vi "Validate move.vi"(7 "Position":refnum<class "Position.lvclass">, 9 "Destination":T1={"File"=enum."d", "Rank"=enum."4"}, 10 "Source":T1={"File"=enum."d", "Rank"=enum."4"}) -> (2 "Valid move":bool, 3 "Move":refnum<class "Move.lvclass">)   [LabVIEW 2016, in "Chesslib.lvlib" / "Move.lvclass"]
uses:
  Move.lvclass
  Pieces/Piece/Piece.lvclass
  Position/Position.lvclass
  typedef/Rank.ctl
  Chesslib.lvlib
  typedef/File.ctl
  typedef/Square.ctl
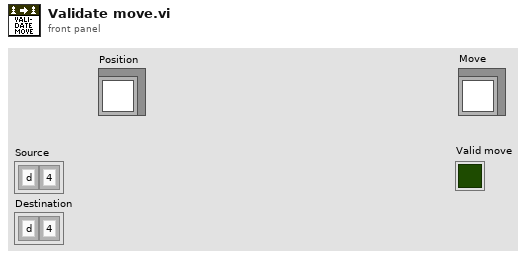
[diagram p1: front panel]
types:
  T1 = typedef "Chesslib.lvlib/Square.ctl" = cluster{"File":T2, "Rank":T3}
  T2 = typedef "Chesslib.lvlib/File.ctl" = enum8{"a", "b", "c", "d", "e", "f", "g", "h"}
  T3 = typedef "Chesslib.lvlib/Rank.ctl" = enum8{"1", "2", "3", "4", "5", "6", "7", "8"}
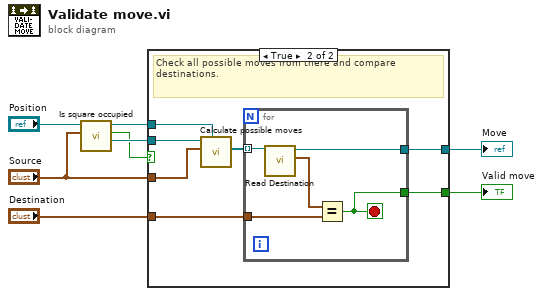
[diagram p0: block diagram]
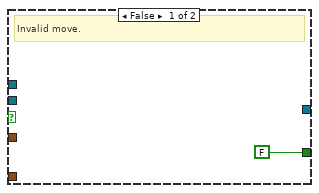
[diagram p2: hidden frame]
diagram:
  n1 = call "Is square occupied.vi"("Square"="Source", "Position in"="Position") -> ("Piece"=w2:refnum<class "Piece.lvclass">, "Occupied"=w1:bool, "Position out"=w4:refnum<class "Position.lvclass">)  [unwired: 6 in, 1 out]
  n2 = case shown="True" w1 {
    tunnel: "Source" -> [_ w16]
    tunnel: "Destination" -> [_ w15]
    tunnel: [_ w14] -> w6
    tunnel: [FALSE w13] -> w5
    tunnel: w4 -> [_ w11]
    tunnel: w2 -> [_ w10]
    frame False {
      # "Invalid move."
    }
    frame True {
      # "Check all possible moves from there and compare destinations."
      n3 = call "Calculate possible moves.vi"("Position"=w11, "Source"=w16, "Piece in"=w10) -> ("Moves"=w12:refnum<class "Move.lvclass">[])  [unwired: 6 in, 2 out]
      n4 = for {
        tunnel: w12 -> [w17] mode=indexing
        tunnel: w15 -> [w21]
        tunnel: [w19] -> w13
        tunnel: [w18] -> w14
        stop <- w19 stop-if-true
        n5 = call "Read Destination.vi"("Move in"=w17) -> ("Square"=w20:T1, "Move out"=w18:refnum<class "Move.lvclass">)  [unwired: 9 in]
        n6 = Equal?(x=w20, y=w21) -> (x = y?=w19:bool)
      }
    }
  }
  "Move" <- w6
  "Valid move" <- w5
